vi "Initialization_UserEvents.vi"(8 "error in":errorcluster, 10 "Layer Clusters":refnum<vi>, 11 "DNL_Framework Templates":refnum<vi>) -> (0 "error out":errorcluster, 2 "User events":T1, 3 "Events":refnum<event-registration>)   [LabVIEW 2020]
doc: "Registers for events and creates User Events related to the Framework Templates and Layers clusters."
uses:
  vi.lib/LabVIEW Icon API/lv_icon/Controls/Graphic.ctl
  Controls/Framework Templates.ctl
  vi.lib/LabVIEW Icon API/lv_icon/Controls/Layer.ctl
  Controls/LayerList.ctl
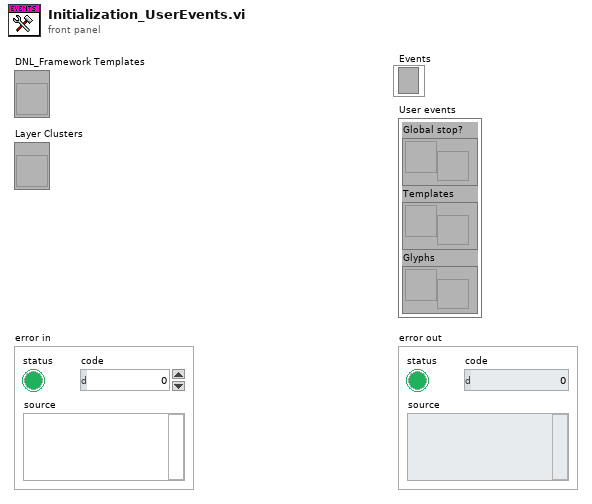
[diagram p1: front panel]
types:
  T1 = cluster{"Global stop?":refnum<user-event>, "Templates":refnum<user-event>, "Glyphs":refnum<user-event>}
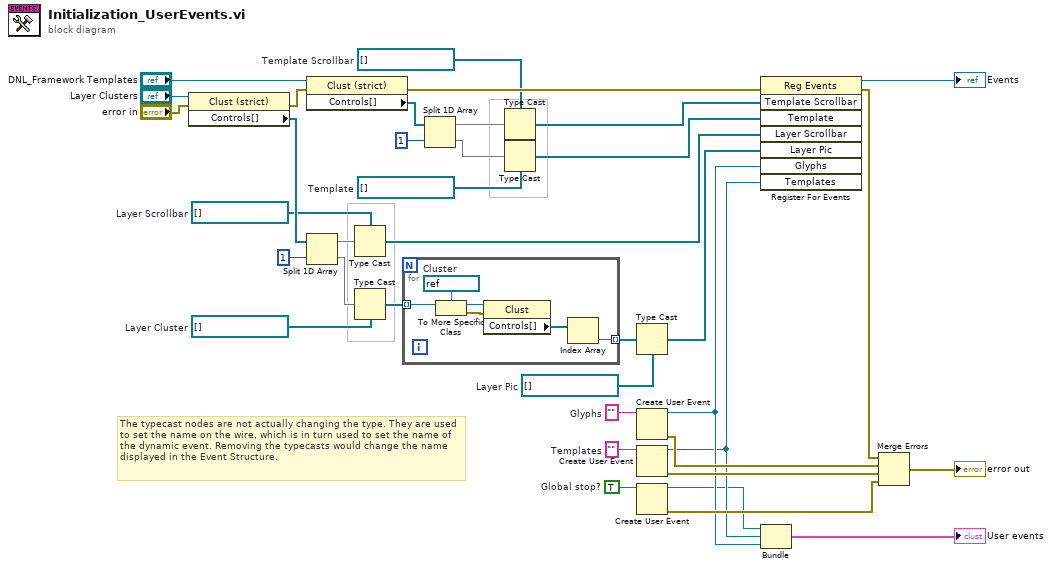
[diagram p0: block diagram]
diagram:
  w8 = TRUE  # Global stop?
  w9 = refnum<vi>[] []  # Template Scrollbar
  w10 = ""  # Templates
  w13 = refnum<vi>[] []  # Layer Pic
  w16 = refnum<vi>[] []  # Layer Scrollbar
  w18 = refnum<vi>[] []  # Template
  w22 = refnum<vi>[] []  # Layer Cluster
  w26 = ""  # Glyphs
  # "The typecast nodes are not actually changing the type. They are used to set the name on the wire, which is in turn used to set the name of the dynamic event. Removing the typecasts would change the name displayed in the Event Structure."
  n1 = property class="Clust (strict)"(reference="Layer Clusters", error in="error in") -> (error out=w36:errorcluster, "Controls[]"=w25:refnum<vi>[])  [unwired: 1 out]
  n2 = property class="Clust (strict)"(reference="DNL_Framework Templates", error in=w36) -> (error out=w37:errorcluster, "Controls[]"=w28:refnum<vi>[])  [unwired: 1 out]
  n3 = Split 1D Array(array=w25, index=1) -> (first subarray=w17:refnum<vi>[], second subarray=w23:refnum<vi>[])
  n4 = Type Cast(type=w16, x=w17) -> (*(type *) &x=w15:refnum<vi>[])
  n5 = Type Cast(type=w22, x=w23) -> (*(type *) &x=w14:refnum<vi>[])
  n6 = for {
    tunnel: w14 -> [w42] mode=indexing
    tunnel: [w38] -> w12 mode=indexing
    w41 = refnum<vi> refnum  # Cluster
    n7 = To More Specific Class(target class=w41, reference=w42) -> (specific class reference=w40:refnum<vi>, error out=w43:errorcluster)  [unwired: 1 in]
    n8 = property class="Clust"(reference=w40, error in=w43) -> ("Controls[]"=w39:refnum<vi>[])  [unwired: 2 out]
    n9 = Index Array(array=w39) -> (element=w38:refnum<vi>)  [unwired: 1 in]
  }
  n10 = Split 1D Array(array=w28, index=1) -> (first subarray=w20:refnum<vi>[], second subarray=w21:refnum<vi>[])
  n11 = Type Cast(type=w9, x=w20) -> (*(type *) &x=w19:refnum<vi>[])
  n12 = Type Cast(type=w18, x=w21) -> (*(type *) &x=w5:refnum<vi>[])
  n13 = Type Cast(type=w13, x=w12) -> (*(type *) &x=w11:refnum<vi>[])
  n14 = Create User Event(user event datatype=w26) -> (user event=w29:refnum<user-event>, error out=w34:errorcluster)  [unwired: 1 in]
  n15 = Create User Event(user event datatype=w10) -> (user event=w7:refnum<user-event>, error out=w33:errorcluster)  [unwired: 1 in]
  n16 = Create User Event(user event datatype=w8) -> (user event=w2:refnum<user-event>, error out=w32:errorcluster)  [unwired: 1 in]
  n17 = register-events(error in=w37, w19, w5, w15, w11, w29, w7) -> (reference out=→"Events":refnum<event-registration>, error out=w31:errorcluster)  [unwired: 1 in]
  n18 = Bundle("Global stop?"=w2, "Templates"=w7, "Glyphs"=w29) -> (→"User events":T1)  [unwired: 1 out]
  n19 = Merge Errors(w31, w34, w33, w32) -> (→"error out":errorcluster)
